vi "set_error_message.vi"(8 "error in (no error)":errorcluster, 10 "error message in":string, 11 "BalloonNotifier in":refnum<class "BalloonNotifier.lvclass">) -> (0 "error out":errorcluster, 3 "BalloonNotifier out":refnum<class "BalloonNotifier.lvclass">)   [LabVIEW 2010, in "BalloonNotifier.lvclass"]
uses:
  BalloonNotifier.lvclass
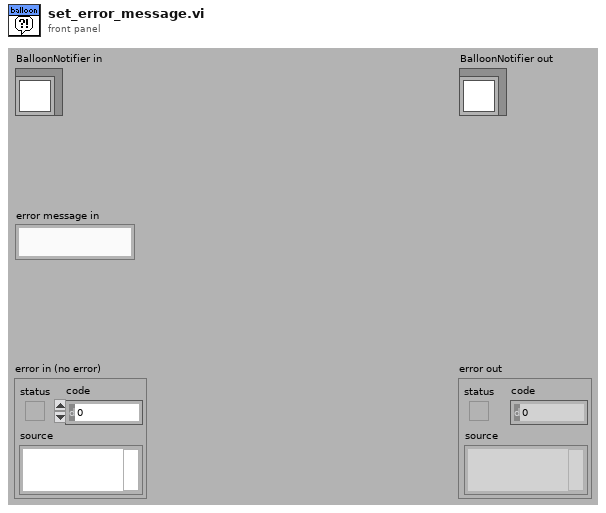
[diagram p1: front panel]
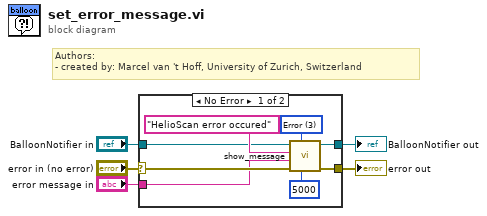
[diagram p0: block diagram]
diagram:
  # "Authors: \n- created by: Marcel van 't Hoff, University of Zurich, Switzerland"
  n1 = case shown="No Error" "error in (no error)" {
    selector: "error in (no error)" -> [w13 w15]
    tunnel: [w7 w15] -> w4
    tunnel: [w8 w14] -> w2
    tunnel: "BalloonNotifier in" -> [w9 w14]
    tunnel: "error message in" -> [w12 _]
    frame No Error {
      w10 = 3 items=["None", "Info", "Warning", "Error"] ("Icon (None)")
      n2 = call-dynamic "show_message.vi"("display time (ms)"=5000, "Icon (None)"=w10, "error in (no error)"=w13, "Text"=w12, "Title"="HelioScan error occured", "BalloonNotifier in"=w9) -> ("error out"=w7:errorcluster, "BalloonNotifier out"=w8:refnum<class "BalloonNotifier.lvclass">)  [unwired: 4 in]
    }
    frame Error {
    }
  }
  "error out" <- w4
  "BalloonNotifier out" <- w2
